vi "Initialize DMM.vi"(6 "initialize and close session behavior":T1, 8 "error in (no error)":errorcluster, 10 "reset":bool, 11 "niDMM in":refnum<class "niDMM.lvclass">) -> (0 "error out":errorcluster, 3 "niDMM out":refnum<class "niDMM.lvclass">)   [LabVIEW 2021, in "niDMM.lvclass"]
doc: "Initializes the driver session for NI-DMM."
uses:
  niDMM.lvclass
  <vilib>/Plug-In SDKs/Clients/Session Management V1/Session Reservation/Initialize and Close Session Behavior.ctl
  niDMM.lvclass/niDMM.ctl
  <vilib>/Plug-In SDKs/Sessions/niDMM/Initialize Sessions - 1Sess.vi
  <vilib>/Plug-In SDKs/Sessions/niDMM/NI Session Management niDMM.lvlib
  <vilib>/Plug-In SDKs/Clients/Session Management V1/Session Reservation/Session Reservation.lvclass
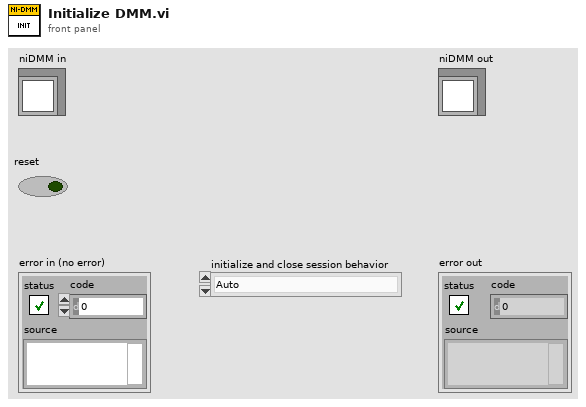
[diagram p1: front panel]
types:
  T1 = typedef "NI Session Management V1 Client.lvlib/Session Reservation.lvclass/Initialize and Close Session Behavior.ctl" = enum16{"Auto", "Initialize and Close", "Attach and Detach", "Initialize and Detach", "Attach and Close"}
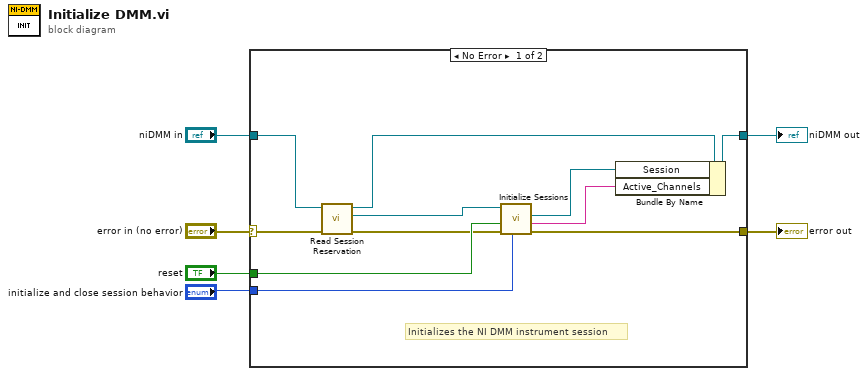
[diagram p0: block diagram]
diagram:
  n1 = case shown="No Error" "error in (no error)" {
    selector: "error in (no error)" -> [w11 w19]
    tunnel: "niDMM in" -> [w8 w18]
    tunnel: [w17 w19] -> w4
    tunnel: [w16 w18] -> w3
    tunnel: "initialize and close session behavior" -> [w13 _]
    tunnel: "reset" -> [w12 _]
    frame No Error {
      # "Initializes the NI DMM instrument session"
      n2 = call-dynamic "Read Session Reservation.vi"("error in (no error)"=w11, "DMM_Base in"=w8) -> ("error out"=w10:errorcluster, "Session Reservation"=w7:refnum<class "Session Reservation.lvclass">, "DMM_Base out"=w9:refnum<class "niDMM.lvclass">)  [unwired: 7 in]
      n3 = call-poly <vilib>:"Initialize Sessions.vi"("initialize and close session behavior"=w13, "error in"=w10, "reset"=w12, "session reservation in"=w7) -> ("error out"=w17:errorcluster, "channel list"=w14:string, "session"=w15:refnum<k15>)  [unwired: 4 in, 1 out]
      n4 = Bundle By Name(cluster=w9, "Session"=w15, "Active_Channels"=w14) -> (w16:refnum<class "niDMM.lvclass">)
    }
    frame Error {
    }
  }
  "error out" <- w4
  "niDMM out" <- w3
